vi "Send to CS.vi"(8 "error in (no error)":errorcluster, 10 "String to write":string, 11 "CS in":refnum<class "CS.lvclass">) -> (0 "error out":errorcluster, 3 "CS out":refnum<class "CS.lvclass">)   [LabVIEW 2013, in "CS.lvclass"]
uses:
  Lib.llb/CS.lvclass
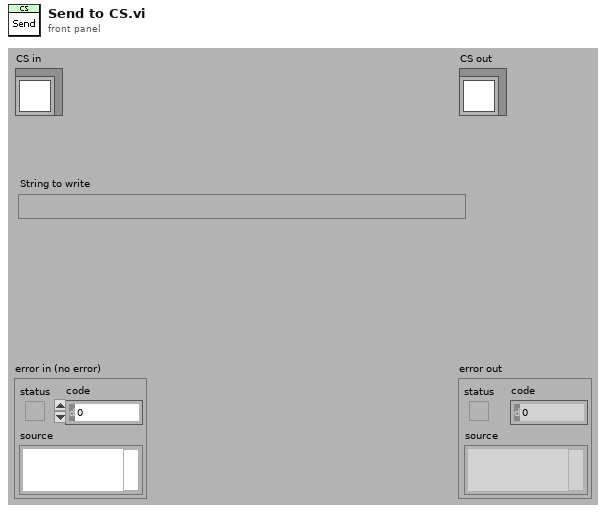
[diagram p1: front panel]
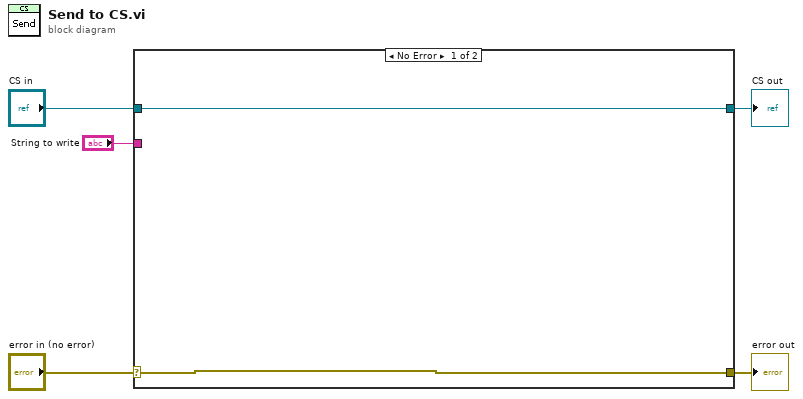
[diagram p0: block diagram]
diagram:
  n1 = case shown="No Error" "error in (no error)" {
    selector: "error in (no error)" -> [w7 w9]
    tunnel: [w7 w9] -> w4
    tunnel: [w6 w8] -> w2
    tunnel: "CS in" -> [w6 w8]
    tunnel: "String to write" -> [_ _]
    frame No Error {
    }
    frame Error {
    }
  }
  "error out" <- w4
  "CS out" <- w2
